vi "调整窗口.vi"(8 "error in (no error)":errorcluster caption="错误输入（无错误）", 10 "前面板范围":T1 caption="窗口范围", 11 "程序 输入":refnum<class "程序.lvclass">) -> (0 "error out":errorcluster caption="错误输出", 3 "程序 输出":refnum<class "程序.lvclass">)   [LabVIEW 2020, in "程序.lvclass"]
uses:
  <vilib>/Utility/miscctls.llb/LVRectTypeDef.ctl
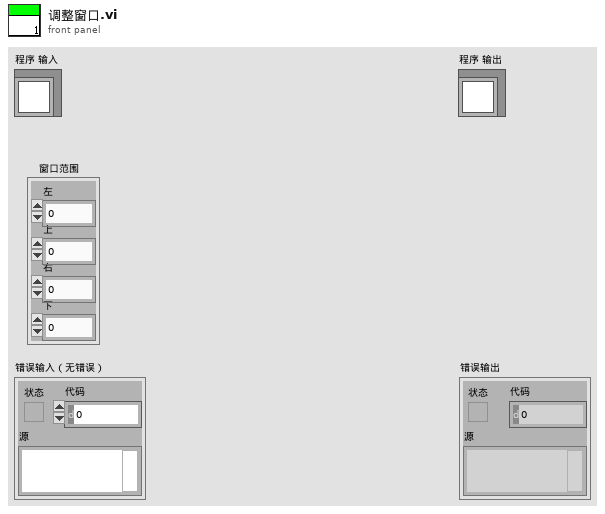
[diagram p1: front panel]
types:
  T1 = typedef "LVRectTypeDef.ctl" = cluster{"Left":i16, "Top":i16, "Right":i16, "Bottom":i16}
  T2 = typedef "LVBoundsTypeDef.ctl" = cluster{"Width":u32, "Height":u32}
  T3 = typedef "LVPositionTypeDef.ctl" = cluster{"Left":i32, "Top":i32}
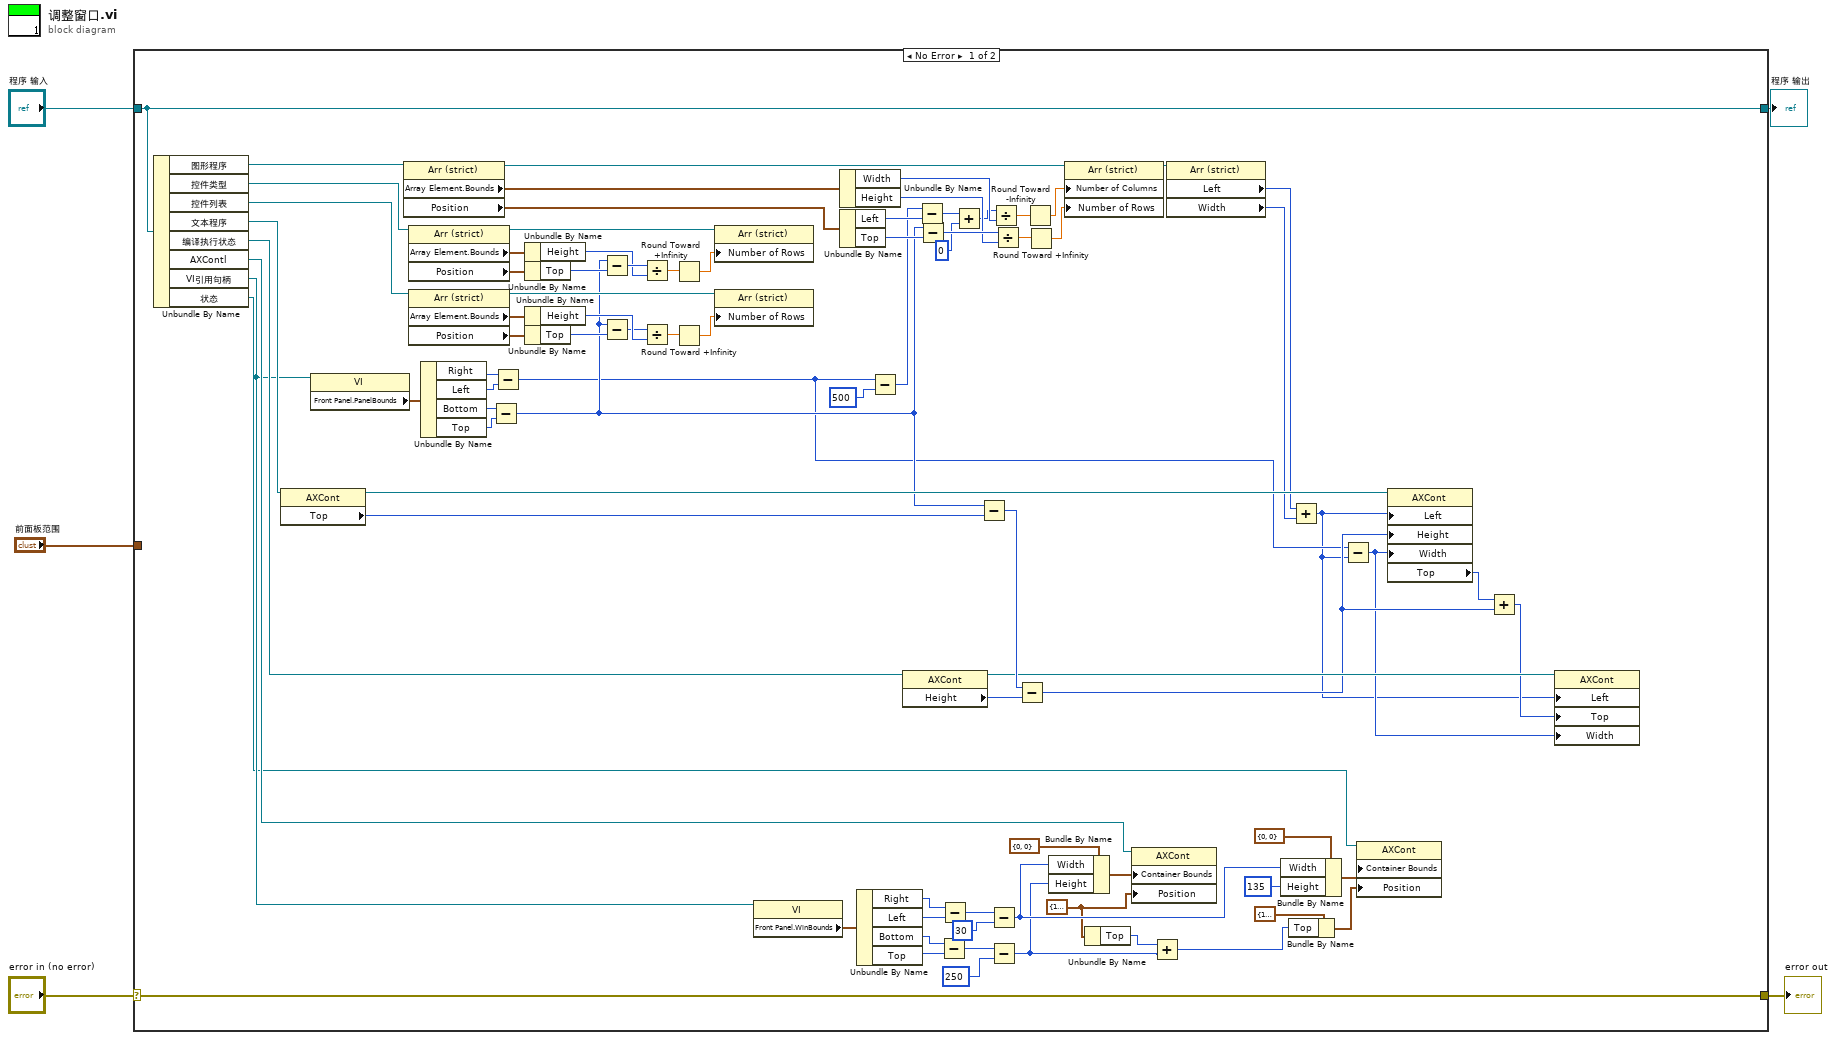
[diagram p0: block diagram]
diagram:
  n1 = case shown="No Error" "error in (no error)" {
    selector: "error in (no error)" -> [w89 w91]
    tunnel: [w89 w91] -> w4
    tunnel: [w88 w90] -> w2
    tunnel: "程序 输入" -> [w88 w90]
    tunnel: "前面板范围" -> [_ _]
    frame No Error {
      w12 = cluster{"Left":i32, "Top":i32} {"Left"=10, "Top"=70} ("位置")
      n2 = Unbundle By Name(w88) -> ("图形程序"=w87:refnum<vi>, "控件类型"=w67:refnum<vi>, "控件列表"=w50:refnum<vi>, "文本程序"=w49:refnum<vi>, "编译执行状态"=w43:refnum<vi>, "AXContl"=w28:refnum<vi>, "VI引用句柄"=w27:refnum<vi>, "状态"=w17:refnum<vi>)
      n3 = property class="AXCont"(reference=w49) -> (reference out=w48:refnum<vi>, "Top"=w45:i32)  [unwired: 1 in, 1 out]
      n4 = property class="VI"(reference=w27) -> ("Front Panel.PanelBounds"=w26:T1)  [unwired: 1 in, 2 out]
      n5 = property class="Arr (strict)"(reference=w87) -> (reference out=w75:refnum<vi>, "Array Element.Bounds"=w79:T2, "Position"=w80:T3)  [unwired: 1 in, 1 out]
      n6 = property class="Arr (strict)"(reference=w67) -> (reference out=w60:refnum<vi>, "Array Element.Bounds"=w66:T2, "Position"=w65:T3)  [unwired: 1 in, 1 out]
      n7 = property class="Arr (strict)"(reference=w50) -> (reference out=w57:refnum<vi>, "Array Element.Bounds"=w51:T2, "Position"=w52:T3)  [unwired: 1 in, 1 out]
      n8 = Unbundle By Name(w26) -> ("Right"=w86:i16, "Left"=w85:i16, "Bottom"=w84:i16, "Top"=w83:i16)
      n9 = Subtract(x=w84, y=w83) -> (x-y=w46:i16)
      n10 = Subtract(x=w86, y=w85) -> (x-y=w21:i16)
      n11 = Unbundle By Name(w66) -> ("Height"=w61:u32)
      n12 = Unbundle By Name(w65) -> ("Top"=w64:i32)
      n13 = Unbundle By Name(w51) -> ("Height"=w56:u32)
      n14 = Unbundle By Name(w52) -> ("Top"=w53:i32)
      n15 = Subtract(x=w46, y=w64) -> (x-y=w62:i32)
      n16 = Subtract(x=w46, y=w53) -> (x-y=w55:i32)
      n17 = Divide(x=w62, y=w61) -> (x/y=w63:dbl)
      n18 = Divide(x=w55, y=w56) -> (x/y=w54:dbl)
      n19 = Round Toward +Infinity(x=w63) -> (ceil(x): smallest int >= x=w59:dbl)
      n20 = Round Toward +Infinity(x=w54) -> (ceil(x): smallest int >= x=w58:dbl)
      n21 = property class="Arr (strict)"(reference=w60, "Number of Rows"=w59) -> ()  [unwired: 1 in, 2 out]
      n22 = property class="Arr (strict)"(reference=w57, "Number of Rows"=w58) -> ()  [unwired: 1 in, 2 out]
      n23 = property class="VI"(reference=w27) -> ("Front Panel.WinBounds"=w39:T1)  [unwired: 1 in, 2 out]
      n24 = Unbundle By Name(w79) -> ("Width"=w78:u32, "Height"=w76:u32)
      n25 = Unbundle By Name(w80) -> ("Left"=w82:i32, "Top"=w81:i32)
      n26 = Unbundle By Name(w39) -> ("Right"=w37:i16, "Left"=w38:i16, "Bottom"=w36:i16, "Top"=w35:i16)
      n27 = Subtract(x=w21, y=i16 500) -> (x-y=w22:i16)
      n28 = property class="AXCont"(reference=w43) -> (reference out=w41:refnum<vi>, "Height"=w42:u32)  [unwired: 1 in, 1 out]
      n29 = Subtract(x=w22, y=w82) -> (x-y=w70:i32)
      n30 = Subtract(x=w46, y=w81) -> (x-y=w77:i32)
      n31 = Subtract(x=w36, y=w35) -> (x-y=w33:i16)
      n32 = Subtract(x=w37, y=w38) -> (x-y=w34:i16)
      n33 = Add(x=w70, y=0) -> (x+y=w69:i32)
      n34 = Subtract(x=w46, y=w45) -> (x-y=w44:i32)
      n35 = Subtract(x=w34, y=i16 30) -> (x-y=w14:i16)
      n36 = Subtract(x=w33, y=i16 250) -> (x-y=w10:i16)
      n37 = Divide(x=w69, y=w78) -> (x/y=w74:dbl)
      n38 = Divide(x=w77, y=w76) -> (x/y=w72:dbl)
      n39 = Subtract(x=w44, y=w42) -> (x-y=w40:u32)
      n40 = Round Toward -Infinity(1:w74) -> (0:w73:dbl)
      n41 = Round Toward +Infinity(x=w72) -> (ceil(x): smallest int >= x=w71:dbl)
      n42 = Bundle By Name(cluster=cluster{"Width":u32, "Height":u32} {"Width"=0, "Height"=0} ("容器边界"), "Width"=w14, "Height"=w10) -> (w30:cluster{"Width":u32, "Height":u32})
      n43 = property class="Arr (strict)"(reference=w75, "Number of Columns"=w73, "Number of Rows"=w71) -> (reference out=w47:refnum<vi>)  [unwired: 1 in, 1 out]
      n44 = Unbundle By Name(w12) -> ("Top"=w11:i32)
      n45 = property on="属性节点" class="AXCont"(reference=w28, "Container Bounds"=w30, "Position"=w12) -> ()  [unwired: 1 in, 2 out]
      n46 = Add(x=w11, y=w10) -> (x+y=w9:i32)
      n47 = property class="Arr (strict)"(reference=w47) -> ("Left"=w20:i32, "Width"=w19:u32)  [unwired: 1 in, 2 out]
      n48 = Bundle By Name(cluster=cluster{"Width":u32, "Height":u32} {"Width"=0, "Height"=0} ("容器边界"), "Width"=w14, "Height"=u32 135) -> (w15:cluster{"Width":u32, "Height":u32})
      n49 = Bundle By Name(cluster=cluster{"Left":i32, "Top":i32} {"Left"=10, "Top"=70} ("位置"), "Top"=w9) -> (w8:cluster{"Left":i32, "Top":i32})
      n50 = Add(x=w20, y=w19) -> (x+y=w6:u32)
      n51 = Subtract(x=w21, y=w6) -> (x-y=w18:u32)
      n52 = property on="属性节点" class="AXCont"(reference=w17, "Container Bounds"=w15, "Position"=w8) -> ()  [unwired: 1 in, 2 out]
      n53 = property class="AXCont"(reference=w48, "Left"=w6, "Height"=w40, "Width"=w18) -> ("Top"=w24:i32)  [unwired: 1 in, 2 out]
      n54 = Add(x=w24, y=w40) -> (x+y=w23:u32)
      n55 = property class="AXCont"(reference=w41, "Left"=w6, "Top"=w23, "Width"=w18) -> ()  [unwired: 1 in, 2 out]
    }
    frame Error {
    }
  }
  "error out" <- w4
  "程序 输出" <- w2
